vi "Acquire.vi"(8 "error in (no error)":errorcluster, 9 "Data Queue":refnum<queue>, 10 "Data Notifier":refnum<notifier>, 11 "Hardware Resources in":T2 {"Baud Rate" items=["<0>"=0, "4800"=4800, "9600"=9600, "19200"=19200, "38400"=38400, "57600"=57600, "115200"=115200]}) -> (0 "error out":errorcluster, 3 "Hardware Resources out":T2 {"Baud Rate" items=["<0>"=0, "4800"=4800, "9600"=9600, "19200"=19200, "38400"=38400, "57600"=57600, "115200"=115200]})   [LabVIEW 2022 SP3, in "Acquisition.lvlib"]
doc: "Perform the acquisition. Replace the contents of this diagram with calls to acquisition hardware."
uses:
  Acquisition.lvlib
  Hardware Configuration.ctl
panel:
  in  "Meas Out":T1
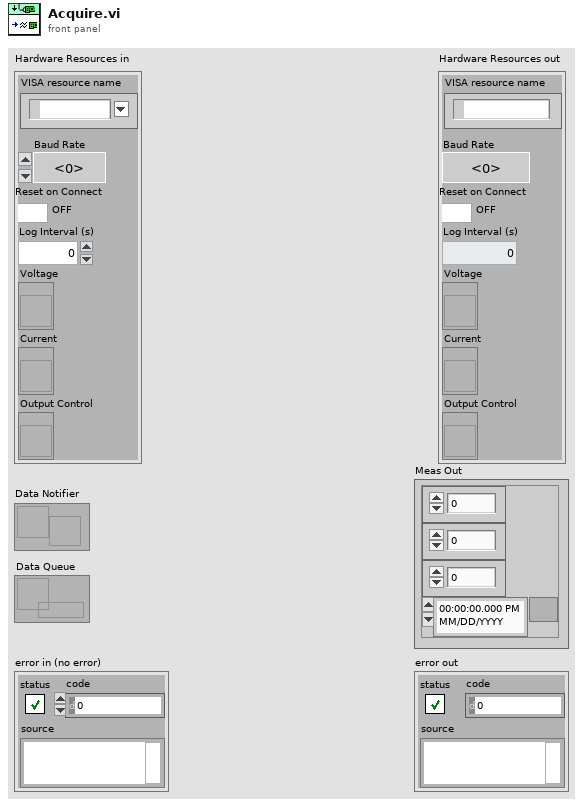
[diagram p1: front panel]
types:
  T1 = cluster{"Voltage":dbl, "Current":dbl, "Power":dbl, timestamp}
  T2 = typedef "Acquisition.lvlib/Hardware Configuration.ctl" = cluster{"VISA resource name":refnum<visa-resource-name>, "Baud Rate":u32, "Reset on Connect":bool, "Log Interval (s)":dbl, "Voltage":refnum<vi>, "Current":refnum<vi>, "Output Control":refnum<vi>}
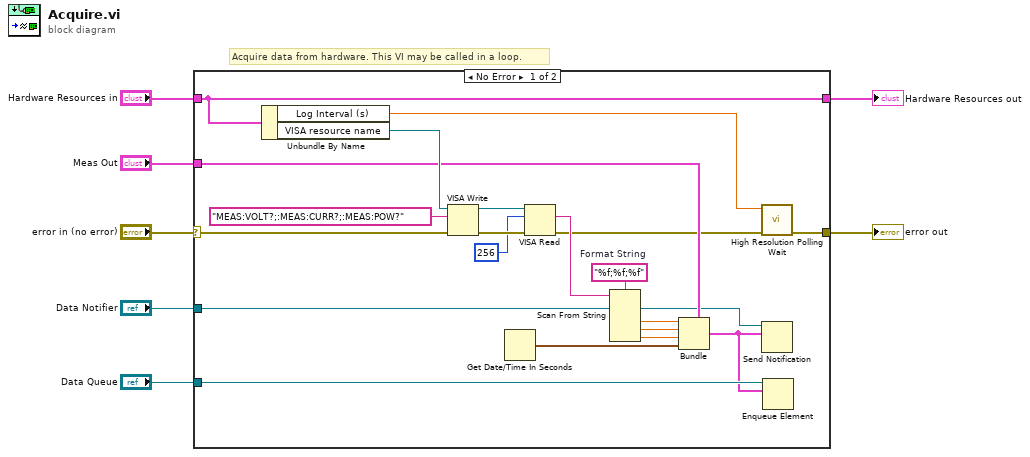
[diagram p0: block diagram]
diagram:
  # "Acquire data from hardware. This VI may be called in a loop."
  n1 = case shown="No Error" "error in (no error)" {
    selector: "error in (no error)" -> [w24 w28]
    tunnel: [w9 w28] -> w6
    tunnel: "Hardware Resources in" -> [w27 w29]
    tunnel: [w27 w29] -> w4
    tunnel: "Meas Out" -> [w16 _]
    tunnel: "Data Notifier" -> [w15 _]
    tunnel: "Data Queue" -> [w14 _]
    frame No Error {
      w21 = "%f;%f;%f"  # Format String
      n2 = Unbundle By Name(w27) -> ("Log Interval (s)"=w8:dbl, "VISA resource name"=w25:refnum<visa-resource-name>)
      n3 = VISA Write(VISA resource name=w25, write buffer="MEAS:VOLT?;:MEAS:CURR?;:MEAS:POW?", error in (no error)=w24) -> (VISA resource name out=w23:refnum<visa-resource-name>, error out=w22:errorcluster)  [unwired: 1 out]
      n4 = Get Date/Time In Seconds() -> (seconds since 1Jan1904=w11:timestamp)
      n5 = VISA Read(VISA resource name=w23, byte count=u32 256, error in (no error)=w22) -> (read buffer=w20:string, error out=w10:errorcluster)  [unwired: 2 out]
      n6 = Scan From String(format string=w21, input string=w20) -> (output 1=w19:dbl, output 2=w18:dbl, output 3=w17:dbl)  [unwired: 5 in, 3 out]
      n7 = Bundle(cluster=w16, "Voltage"=w19, "Current"=w18, "Power"=w17, w11) -> (w13:T1)
      n8 = call <vilib>:"High Resolution Polling Wait.vi"("error in (no error)"=w10, "seconds to wait"=w8) -> ("error out"=w9:errorcluster)  [unwired: 9 in]
      n9 = Send Notification(notification=w13, notifier=w15) -> ()  [unwired: 1 in, 2 out]
      n10 = Enqueue Element(queue=w14, element=w13) -> ()  [unwired: 2 in, 3 out]
    }
    frame Error {
    }
  }
  "Hardware Resources out" <- w4
  "error out" <- w6
